vi "add to log.vi"(0 "Path":path, 9 "User-data cluster":T3, 11 "error in (no error)":errorcluster, 12 "Data":string) -> (15 "error out":errorcluster)   [LabVIEW 2012]
uses:
  typedef/User_Data_Cluster.ctl
  typedef/User Accounts.ctl
  typedef/Log_User_Data.ctl
panel:
  out "output cluster":T1
  in  "Log\n User-data cluster":T1
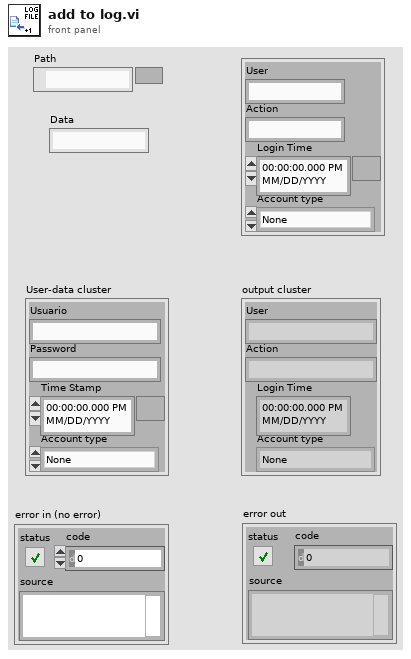
[diagram p1: front panel]
types:
  T1 = typedef "Log_User_Data.ctl" = cluster{"User":string, "Action":string, "Account type":T2, "Login Time ":timestamp}
  T2 = typedef "User Accounts.ctl" = enum16{"None", "User", "Admin"}
  T3 = typedef "User_Data_Cluster.ctl" = cluster{"Usuario":string, "Password":string, "Account type":T2, "Time Stamp":timestamp}
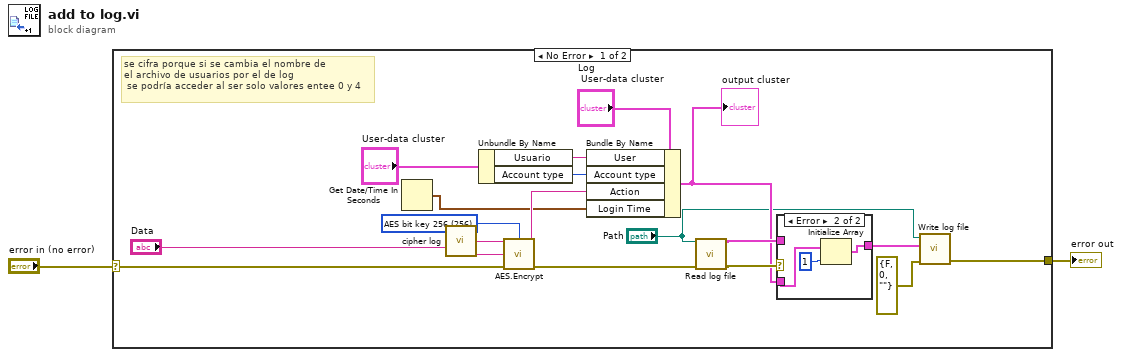
[diagram p0: block diagram]
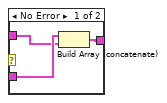
[diagram p2: hidden frame]
diagram:
  n1 = case shown="No Error" "error in (no error)" {
    selector: "error in (no error)" -> [w15 w27]
    tunnel: [w5 w27] -> w1
    frame No Error {
      w17 = u16 256 items=["AES bit key 128"=128, "AES bit key 192"=192, "AES bit key 256"=256] ("BitKeyType(256)")
      # "se cifra porque si se cambia el nombre de\nel archivo de usuarios por el de log\n se podría acceder al ser solo valores entee 0 y 4"
      n2 = Get Date/Time In Seconds() -> (seconds since 1Jan1904=w12:timestamp)
      n3 = call "cipher log.vi"() -> ("password to cipher log"=w16:string)  [unwired: 15 in]
      n4 = Unbundle By Name("User-data cluster") -> ("Usuario"=w18:string, "Account type"=w19:T2)
      n5 = call <vilib>:"AES.Encrypt.vi"("Password"=w16, "BitKeyType (256)"=w17, "PlainText"="Data", "error in"=w15) -> ("CypheredText"=w20:string, "error out"=w8:errorcluster)  [unwired: 10 in]
      n6 = Bundle By Name(cluster="Log\n User-data cluster", "User"=w18, "Account type"=w19, "Action"=w20, "Login Time"=w12) -> (w7:T1)
      "output cluster" <- w7
      n7 = call "Read log file.vi"("file path (use dialog)"="Path", "error in"=w8) -> ("Array"=w9:T1[], "error out"=w10:errorcluster)  [unwired: 12 in]
      n8 = case shown="Error" w10 {
        tunnel: w9 -> [w21 _]
        tunnel: [w23 w24] -> w11
        tunnel: w7 -> [w22 w25]
        frame No Error {
          n9 = Build Array (concatenate)(w22, w21) -> (w23:T1[])
        }
        frame Error {
          n10 = Initialize Array(w25, 1 ("dimension size")) -> (w24:T1[])
        }
      }
      n11 = call "Write log file.vi"("error in"=errorcluster {"status"=FALSE, "code"=0, "source"=""}, "UDcluster Array in"=w11, "file path (use dialog)"="Path") -> ("error out"=w5:errorcluster)  [unwired: 7 in, 1 out]
    }
    frame Error {
    }
  }
  "error out" <- w1
